vi "Trav_pos_global.vi"() -> ()   [LabVIEW 2021]
uses:
  Gen Trav/Traverse_cluster.ctl
  Gen Trav/Spacing.ctl
  Controls/Multi_run_mode.ctl
  Controls/Tunnel_Coordinates.ctl
  Controls/PP Raw data file cluster.ctl
  Controls/GMU Gas Line Name.ctl
  Gen Trav/Route mapping/Exclude_cluster.ctl
  Gen Trav/Route mapping/Box_size.ctl
  Gen Trav/Route mapping/Exclusion_type.ctl
panel:
  in  "Tab Control":T1(tab)
  in  "pointID":string
  in  "Current Row":T2 {"Carrier_2 Q (l/min)" format="%#.2f"; "Row Duration (mins)" format="%#.1f"; "Row No" min=0; "Trace Gas Concentration (%)" min=0.0 format="%#_4f"; "Carrier_1 Q (l/min)" format="%#.4f"; "Start X" format="%#.2f"; "Start Y" format="%#.2f"; "Start Z" format="%#.2f"; "End X" format="%#.2f"; "End Y" format="%#.2f"; "End Z" format="%#.2f"; "Tunnel Speed" format="%#.2f"; "Averaging time (mins)" min=0.0 format="%#.2f"}
  out "Currently on point":i32=9
  in  "Paused During Row?":bool
  out "Axis Traversed":enum16{"X traverse", "Y traverse", "Z traverse"}(ring)
  in  "MultiRun Has Jumped?":bool
  in  "Traverse position":sgl[](array[numeric])=[0.0, 0.0, 0.0] format="%.2f"
  in  "Live Position":sgl[](array[numeric])=[0.0, 0.0, 0.0] format="%.6f"
  in  "Live Channel Position":sgl[](array[numeric])=[0.0, 0.0, 0.0] format="%.6f"
  in  "Traverse Origin X Offset (mm)":sgl min=0 max=20000
  in  "Traverse position Offset":sgl[](array[numeric])=[0.0, 0.0, 0.0] format="%.2f"
  in  "Trav_Coordinates Current Pos dx;dy;dz":sgl[](array[numeric])=[0.0, 0.0, 0.0] format="%.2f"
  in  "3D Live Position Offset":sgl[](array[numeric])=[0.0, 0.0, 0.0] format="%.2f"
  in  "UW Offset Position (Tun Cord)":sgl[](array[numeric])=[0.0, 0.0, 0.0] format="%.2f"
  in  "UW Offset Traverse Name":string
  in  "Work in Tunnel Coordinates?":T5
  in  "Mirror Up?":bool=TRUE
  in  "Speed Factor":sgl=1.0 min=0.1 max=60 format="%.2f"
  in  "Traverse Output Board Number":u32=1
  in  "Maximum Step Size (mm) for checking Trajectory":sgl=100.0
  in  "Minimum Step Size (mm) for checking Trajectory":sgl=10.0
  in  "Default Traverse Setup":string
  in  "Traverse Computer IP Number":string
  out "Live Traverse Preview?":bool
  in  "Fast Plotting?":bool
  in  "Multi_Run_Prog_Start_Time":dbl
  in  "Start of Row time (Sec)":dbl
  out "Trav Last Moved":timestamp
  out "Row completion times":timestamp[](array[timestamp])
  out "Simulation Time":timestamp
  in  "Pause Until Seconds 1904":dbl
  in  "Estimated Completion time":string
  in  "Cmd File Prefix":string
  in  "Results File Prefix":string
  in  "Pause Acquisition":bool
  in  "Dummy Measurement?":bool
  in  "Measurement setup files":string[](array[string])
  in  "Meas Setup Number":i32
  in  "Current Meas Setup File":string
  in  "Top level setup filename":path
  in  "Current Image Filename":path
  out "Raw Data filenames to Post Process":T6[](array[typedef])
  in  "Default Gas Line Name":T7
  in  "FFID Background":T2 {"Carrier_2 Q (l/min)" format="%#.2f"; "Row Duration (mins)" format="%#.1f"; "Row No" min=0; "Trace Gas Concentration (%)" min=0.0 format="%#_4f"; "Carrier_1 Q (l/min)" format="%#.4f"; "Start X" format="%#.2f"; "Start Y" format="%#.2f"; "Start Z" format="%#.2f"; "End X" format="%#.2f"; "End Y" format="%#.2f"; "End Z" format="%#.2f"; "Tunnel Speed" format="%#.2f"; "Averaging time (mins)" min=0.0 format="%#.2f"}
  in  "Bkgnd Number Since Calibration":i32
  in  "Sync to server now":bool
  in  "Source Control?":bool
  in  "Multi Run has Inlet Heaters Enabled?":bool
  in  "Route checking Chs":string[](array[string])
  in  "ADAM Positions Ch names":string[](array[string])
  in  "Traverses to Move":string[](array[string])
  in  "Show User Metadata on Launch?":bool=TRUE
  out "ADAM Channels in Model Coordinates":string[](array[string])
  out "Exclude Array":T8[](array[typedef]) {"Sizes"."Min" format="%#.1f"; "Sizes"."Max" format="%#.1f"}
  # "X           Y          Z"
  # "Start"
  # "End"
  # "X                Y                   Z"
  # "X           Y          Z"
  # "Start"
  # "End"
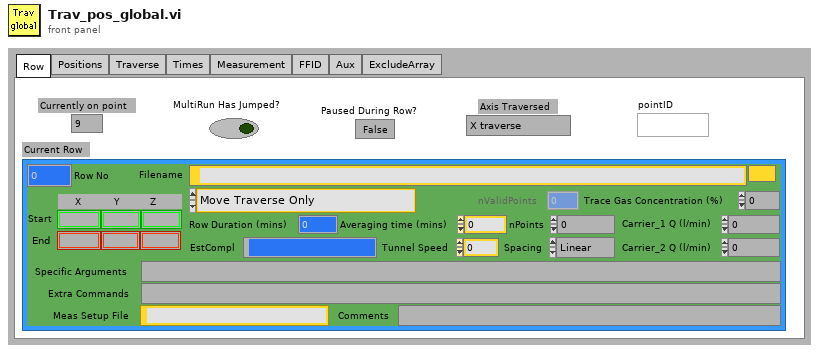
[diagram p1: front panel]
types:
  T1 = enum32{"Row", "Positions", "Traverse", "Times", "Measurement", "FFID", "Aux", "ExcludeArray"}
  T2 = typedef "Traverse_cluster.ctl" = cluster{"Start X":sgl, "Start Y":sgl, "Start Z":sgl, "End X":sgl, "End Y":sgl, "End Z":sgl, "nPoints":i32, "Spacing":T3, "Filename":path, "Tunnel Speed":dbl, "Averaging time (mins)":dbl, "Extra Commands":string, "Carrier_1 Q (l/min)":dbl, "Carrier_2 Q (l/min)":dbl, "Trace Gas Concentration (%)":dbl, "Specific Arguments":string, "Comments":string, "Row No":i32, "Row Type Selector":T4, "EstCompl":string, "Row Duration (mins)":dbl, "nValidPoints":i32, "Meas Setup File":string}
  T3 = typedef "Spacing.ctl" = enum16{"Linear", "Log", "Gauss", "Specified", "N/A"}
  T4 = typedef "Multi_run_mode.ctl" = enum16{"Move Traverse Only", "Set Tunnel Speed Only", "Set Source Only", "Set Measurement Conditions", "Single Measurement", "Vertical Profile", "Lateral Profile", "Longitudinal Profile", "Multi-Axis Profile", "Explore Volume", "Auto Calibrate", "Meas Fast FID Bkgnd", "Check Beam Power", "Scanning Valve Measurement", "Run VI Named:", "Set ADAM Ch", "Wait (minutes)", "Send Message", "Synchronize With:", "Fall Back to this Row", "Turn Off Row Repeating", "Traverse 3D Volume", "Blank Row", "Jump to Fall Back Row"}
  T5 = typedef "Tunnel_Coordinates.ctl" = enum16{"Work in Tunnel Coordinates", "Work in Model Coordinates"}
  T6 = typedef "PP Raw data file cluster.ctl" = cluster{"Raw Data File":path, "Results File":path}
  T7 = typedef "GMU Gas Line Name.ctl" = enum16{"GMU1 Source", "GMU2 Source", "GMU2 Calib", "CPP GRC-A", "CPP GRC-B"}
  T8 = typedef "Exclude_cluster.ctl" = cluster{"Sizes":T9, "Name":string, "Exclude Type":T10}
  T9 = typedef "Box_size.ctl" = cluster{"Max":sgl, "Min":sgl}[]
  T10 = typedef "Exclusion_type.ctl" = enum16{"Exclude completely", "Allow only vertical moves"}
diagram:
